vi "Calculate DNL - Histogram.vi"(11 "histogram":i32[](array[numeric])) -> (3 "DNL":dbl[](array[numeric]))   [LabVIEW 2021]
uses:
  <vilib>/Analysis/baseanly.llb/Mean (DBL).vi
  <vilib>/Analysis/NI_AALBase.lvlib
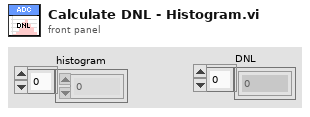
[diagram p1: front panel]
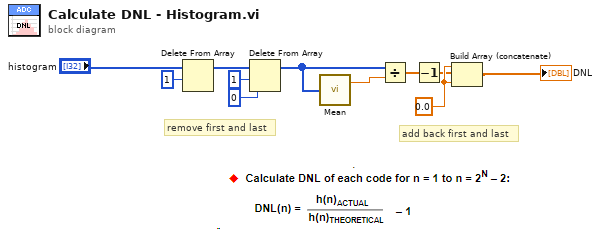
[diagram p0: block diagram]
diagram:
  w10 = 0.0
  # "add back first and last"
  # "remove first and last"
  n1 = Delete From Array(array="histogram", length=1) -> (array with subset deleted=w4:i32[])  [unwired: 1 in, 1 out]
  n2 = Delete From Array(array=w4, length=1, index=0) -> (array with subset deleted=w6:i32[])  [unwired: 1 out]
  n3 = call-poly <vilib>:"Mean.vi"("X"=w6) -> ("mean"=w7:dbl)  [unwired: 1 out]
  n4 = Divide(x=w6, y=w7) -> (x/y=w8:dbl[])
  n5 = Decrement(x=w8) -> (x-1=w9:dbl[])
  n6 = Build Array (concatenate)(w10, w9, w10) -> (→"DNL":dbl[])
